vi "ReadInput.vi"(11 "Enter initials":string) -> (1 "all rows 3":dbl[][](array[numeric]), 2 "all rows 2":dbl[][](array[numeric]), 3 "all rows":dbl[][](array[numeric]))   [LabVIEW 2018]
uses:
  <vilib>/Utility/file.llb/Read Delimited Spreadsheet (DBL).vi
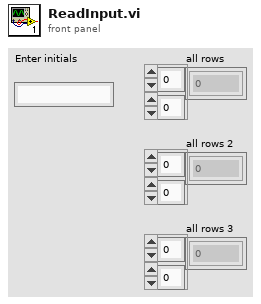
[diagram p1: front panel]
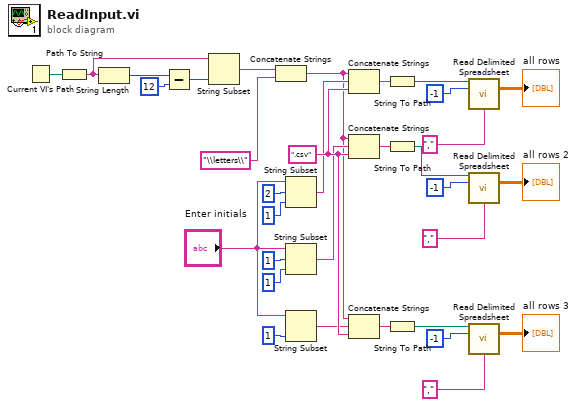
[diagram p0: block diagram]
diagram:
  w18 = ".csv" ("string")
  n1 = Current VI's Path() -> (path=w6:path)
  n2 = Path To String(path=w6) -> (string=w2:string)
  n3 = String Length(string=w2) -> (length=w5:i32)
  n4 = Subtract(x=w5, y=12) -> (x-y=w3:i32)
  n5 = String Subset(string=w2, length (rest)=w3) -> (substring=w1:string)  [unwired: 1 in]
  n6 = Concatenate Strings(w1, "\\letters\\" ("string")) -> (w7:string)
  n7 = String Subset(string="Enter initials", offset (0)=2, length (rest)=1 ("length (rest)")) -> (substring=w17:string)
  n8 = String Subset(string="Enter initials", offset (0)=1, length (rest)=1 ("length (rest)")) -> (substring=w16:string)
  n9 = String Subset(string="Enter initials", length (rest)=1 ("length (rest)")) -> (substring=w15:string)  [unwired: 1 in]
  n10 = Concatenate Strings(w7, w17, w18) -> (w30:string)
  n11 = Concatenate Strings(w7, w16, w18) -> (w32:string)
  n12 = Concatenate Strings(w7, w15, w18) -> (w29:string)
  n13 = String To Path(string=w30) -> (path=w31:path)
  n14 = String To Path(string=w32) -> (path=w33:path)
  n15 = String To Path(string=w29) -> (path=w28:path)
  n16 = call-poly <vilib>:"Read Delimited Spreadsheet.vi"("file path (dialog if empty)"=w31, "number of rows (all:-1)"=-1, "delimiter (\\t)"="," ("delimiter (\\t)")) -> ("all rows"=→"all rows":dbl[][])  [unwired: 7 in, 5 out]
  n17 = call-poly <vilib>:"Read Delimited Spreadsheet.vi"("file path (dialog if empty)"=w33, "number of rows (all:-1)"=-1, "delimiter (\\t)"="," ("delimiter (\\t)")) -> ("all rows"=→"all rows 2":dbl[][])  [unwired: 7 in, 5 out]
  n18 = call-poly <vilib>:"Read Delimited Spreadsheet.vi"("file path (dialog if empty)"=w28, "number of rows (all:-1)"=-1, "delimiter (\\t)"="," ("delimiter (\\t)")) -> ("all rows"=→"all rows 3":dbl[][])  [unwired: 7 in, 5 out]
